vi "Funnel_Set.vi"() -> ()   [LabVIEW 2020]
uses:
  Funnel_Cluster.ctl
  Control_States_Funnel.ctl
  Globals/Funnel_global.vi
panel:
  in  "deadzone":dbl
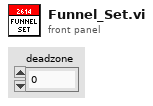
[diagram p1: front panel]
types:
  T1 = typedef "Control_States_Funnel.ctl" = enum16{"No_Op", "Manual_Op"}
  T2 = typedef "Funnel_Cluster.ctl" = cluster{"Control States":T1, "Throttle":dbl}
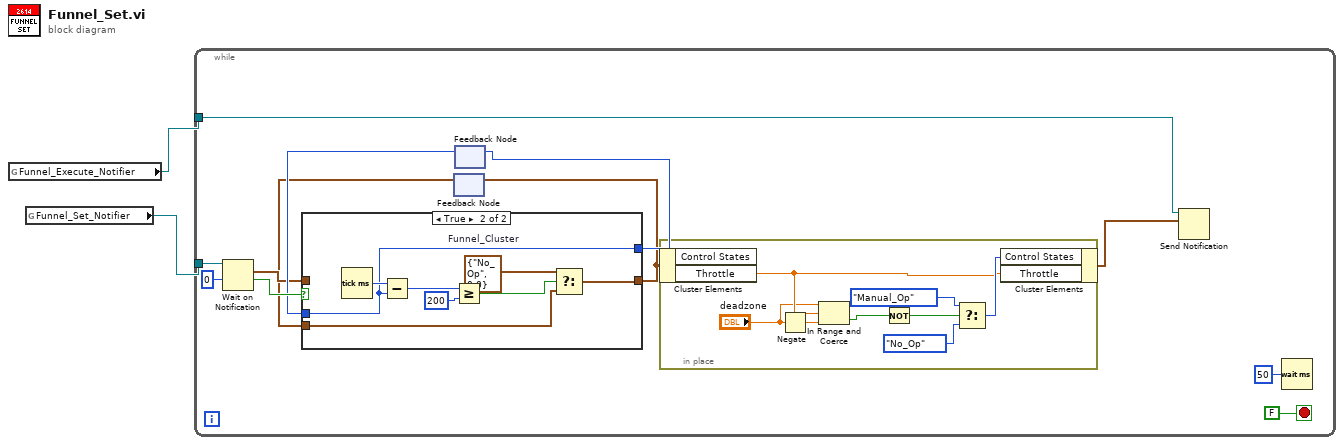
[diagram p0: block diagram]
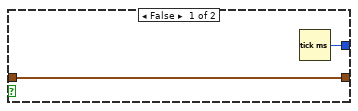
[diagram p2: hidden frame]
diagram:
  n1 = global read "Funnel_global.vi" "Funnel_Execute_Notifier"() -> (w2:refnum<notifier>)
  n2 = global read "Funnel_global.vi" "Funnel_Set_Notifier"() -> (w1:refnum<notifier>)
  n3 = while {
    tunnel: w1 -> [w6]
    tunnel: w2 -> [w3]
    stop <- FALSE stop-if-true
    n4 = Wait on Notification(notifier=w6, timeout in ms (-1)=0) -> (notification=w8:T2, timed out?=w11:bool)  [unwired: 2 in, 2 out]
    n5 = feedback #1() -> (w7:T2)  [unwired: 1 in]
    n6 = feedback #2() -> (w9:u32)  [unwired: 1 in]
    n7 = case shown="True" w11 {
      tunnel: w8 -> [w24 _]
      tunnel: [w24 w32] -> w5
      tunnel: w7 -> [_ w31]
      tunnel: [w23 w29] -> w10
      tunnel: w9 -> [_ w29]
      frame False {
        n8 = Tick Count (ms)() -> (millisecond timer value=w23:u32)
      }
      frame True {
        w25 = T2 {"Control States"=enum."No_Op", "Throttle"=0.0}  # Funnel_Cluster
        n9 = Tick Count (ms)() -> (millisecond timer value=w30:u32)
        n10 = Subtract(x=w30, y=w29) -> (x-y=w27:u32)
        n11 = Greater Or Equal?(x=w27, y=u32 200) -> (x >= y?=w28:bool)
        n12 = Select(t=w25, s=w28, f=w31) -> (s? t:f=w32:T2)
      }
    }
    n13 = feedback-in #1(w5) -> ()
    n14 = feedback-in #2(w10) -> ()
    n15 = in-place {
      n16 = in-place-cluster #3(w5) -> ("Throttle"=w19:dbl)  [unwired: 1 out]
      n17 = Negate(x="deadzone") -> (-x=w17:dbl)
      n18 = In Range and Coerce(upper limit="deadzone", x=w19, lower limit=w17) -> (In Range?=w16:bool)  [unwired: 1 out]
      n19 = Not(x=w16) -> (.not. x?=w15:bool)
      n20 = Select(t=Control_States_Funnel."Manual_Op" ("Control States"), s=w15, f=Control_States_Funnel."No_Op" ("Control States")) -> (s? t:f=w20:T1)
      n21 = in-place-cluster #3("Control States"=w20, "Throttle"=w19) -> (w4:T2)
    }
    n22 = Send Notification(notification=w4, notifier=w3) -> ()  [unwired: 1 in, 2 out]
    n23 = Wait (ms)(milliseconds to wait=u32 50) -> ()  [unwired: 1 out]
  }
